vi "ASTI FREQ CALC v3.1 .vi"(8 "Calculate":bool, 9 "Path":u16(ring) items=["AMC 8 PRI : 7(A)", "AMC 8 PRI : 9(B)", "G13 ALT : 17(A)", "G13 ALT : 1(B)"], 10 "Input Frequency (MHz)":dbl=70.0 format="%.4g") -> (1 "C-band RX":dbl format="%.4g", 2 "C-Band TX":dbl format="%.4g")   [LabVIEW 2015]
uses:
  <vilib>/printing/EasyPrintingControls.llb/contents.ctl
  <vilib>/printing/EasyPrintingControls.llb/layout_options.ctl
  <vilib>/printing/EasyPrintingControls.llb/orientation.ctl
  <vilib>/printing/EasyPrintingControls.llb/panel_scaling_for_page.ctl
  <vilib>/printing/EasyPrintingControls.llb/margins.ctl
  <vilib>/printing/EasyPrintingControls.llb/margin_values.ctl
  <vilib>/printing/EasyPrintingControls.llb/measurement_system.ctl
  <vilib>/printing/EasyPrintingControls.llb/printer_options.ctl
  <vilib>/printing/EasyPrintingControls.llb/printing_method.ctl
  <vilib>/printing/EasyPrintingControls.llb/color_or_monochrome.ctl
  <vilib>/printing/EasyPrintingControls.llb/page_header_options.ctl
  <vilib>/printing/EasyPrintingControls.llb/page_headers.ctl
  <vilib>/printing/EasyPrintingControls.llb/page_header_content_options.ctl
  <vilib>/printing/EasyPrintingControls.llb/report_type.ctl
  <vilib>/Utility/file.llb/Read Delimited Spreadsheet (string).vi
  <vilib>/printing/EasyPrinting.llb/Easy Print VI Panel or Documentation (path).vi
  <vilib>/Utility/NIReport.llb/NI_ReportGenerationCore.lvlib
panel:
  in  "Print":bool
  out "TIME":string
  out "DATE":string
  out "Status":string
  in  "stop":bool
  in  "Tab Control":T1(tab)
  in  "Direction (L-Band Only)":u16(ring) items=["L-Band TX", "L-Band RX"]
  in  "Add to report":bool
  out "Frequency Ranges (Center)":string[][](array[string])
  out "70 2":dbl format="%.4g"
  out "70":dbl format="%.4g"
  out "L-RX":dbl format="%.4g"
  out "L-TX":dbl format="%.4g"
  in  "Clear":bool
  in  "Carrier":string[][](array[string])=[["Carrier/Link", "C-Band TX            ", "C-Band RX       ", "L-Band TX       ", "L-Band RX       ", "70MHz-IF     "], ["", "3840.000000", "1165.000000", "1310.000000", "70.000000", ""], ["", "0.000000", "0.000000", "0.000000", "0.000000", ""], ["", "3840.000000", "1165.000000", "1310.000000", "70.000000", ""], ["", "", "", "", "", ""], ["", "", "", "", "", ""], ["", "", "", "", "", ""], ["", "", "", "", "", ""], ["", "     ", "", "       ", "", ""], ["", "        ", "", "        ", "", ""]]
  out "Frequencies":string[][](array[string])=[["C-Band TX            ", "C-Band RX       ", "L-Band TX       ", "L-Band RX       ", "70MHz-IF     ", ""], ["", "", "", "", "", ""], ["", "", "", "", "", ""], ["", "", "", "", "", ""], ["", "", "", "", "", ""], ["", "", "", "", "", ""], ["", "     ", "", "       ", "", ""], ["", "        ", "", "        ", "", ""]]
  in  "Site":string
  # "ASTI FREQUENCY CALC"
  # "Transmit IF"
  # "70MHz"
  # "RF\nEquip"
  # "Transmitting\nModem"
  # "Or"
  # "L-Band"
  # "BUC LO = 4900"
  # "LO = 2225 MHz"
  # "All frequency values are in MHz"
  # "Sat"
  # "Receive IF"
  # "70MHz"
  # "RF\nEquip"
  # "Receiving\nModem"
  # "Or"
  # "Note: Downlink C-Band frequencies are not accessible at sites with L-Band IF\nIF/RF Equipment"
  # "L-Band"
  # "LNB LO = 5150"
  # "** Converters and modems are configured with 20 MHz offset at 70MHz-IF and converter CF"
  # "Edit carrier name\nprior to printing"
  # "For a single carrier"
  # "(LBand TX)  +  LBand RX = 2475 MHz"
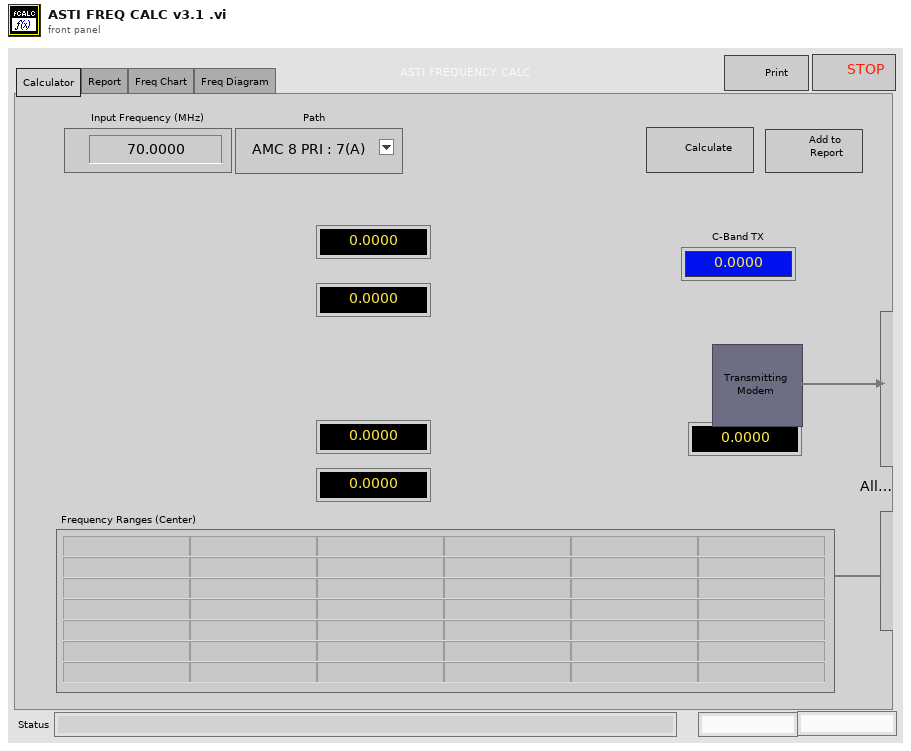
[diagram p1: front panel]
types:
  T1 = enum32{"Calculator", "Report", "Freq Chart", "Freq Diagram"}
  T2 = cluster{"C-Band TX":dbl, "C-band RX":dbl, "L-TX":dbl, "L-RX":dbl, "70":dbl}
  T3 = typedef "NI_ReportGenerationCore.lvlib/layout_options.ctl" = cluster{"orientation (unchanged)":T4, "panel scaling for page (unchanged)":T5, "margins":T6, "printer options":T9, "page header options":T12}
  T4 = typedef "NI_ReportGenerationCore.lvlib/orientation.ctl" = u16
  T5 = typedef "NI_ReportGenerationCore.lvlib/panel_scaling_for_page.ctl" = u16
  T6 = typedef "NI_ReportGenerationCore.lvlib/margins.ctl" = cluster{"override VI margins (false)":bool, "margins (1.00)":T7, "measurement system (default)":T8}
  T7 = typedef "NI_ReportGenerationCore.lvlib/margin_values.ctl" = cluster{"top":dbl, "left":dbl, "right":dbl, "bottom":dbl}
  T8 = typedef "NI_ReportGenerationCore.lvlib/measurement_system.ctl" = u16
  T9 = typedef "NI_ReportGenerationCore.lvlib/printer_options.ctl" = cluster{"destination printer name (current)":string, "printing method (unchanged)":T10, "color or monochrome (unchanged)":T11}
  T10 = typedef "NI_ReportGenerationCore.lvlib/printing_method.ctl" = u16
  T11 = typedef "NI_ReportGenerationCore.lvlib/color_or_monochrome.ctl" = u16
  T12 = typedef "NI_ReportGenerationCore.lvlib/page_header_options.ctl" = cluster{"page headers (unchanged)":T13, "page header content options":T14}
  T13 = typedef "NI_ReportGenerationCore.lvlib/page_headers.ctl" = u16
  T14 = typedef "NI_ReportGenerationCore.lvlib/page_header_content_options.ctl" = cluster{"Include VI Name":bool, "Include VI Path":bool, "Include Last Modification Date":bool, "Include Date Printed":bool, "Include Page Number":bool, "Include VI Icon":bool}
  T15 = typedef "NI_ReportGenerationCore.lvlib/report_type.ctl" = u16
  T16 = typedef "NI_ReportGenerationCore.lvlib/contents.ctl" = u16
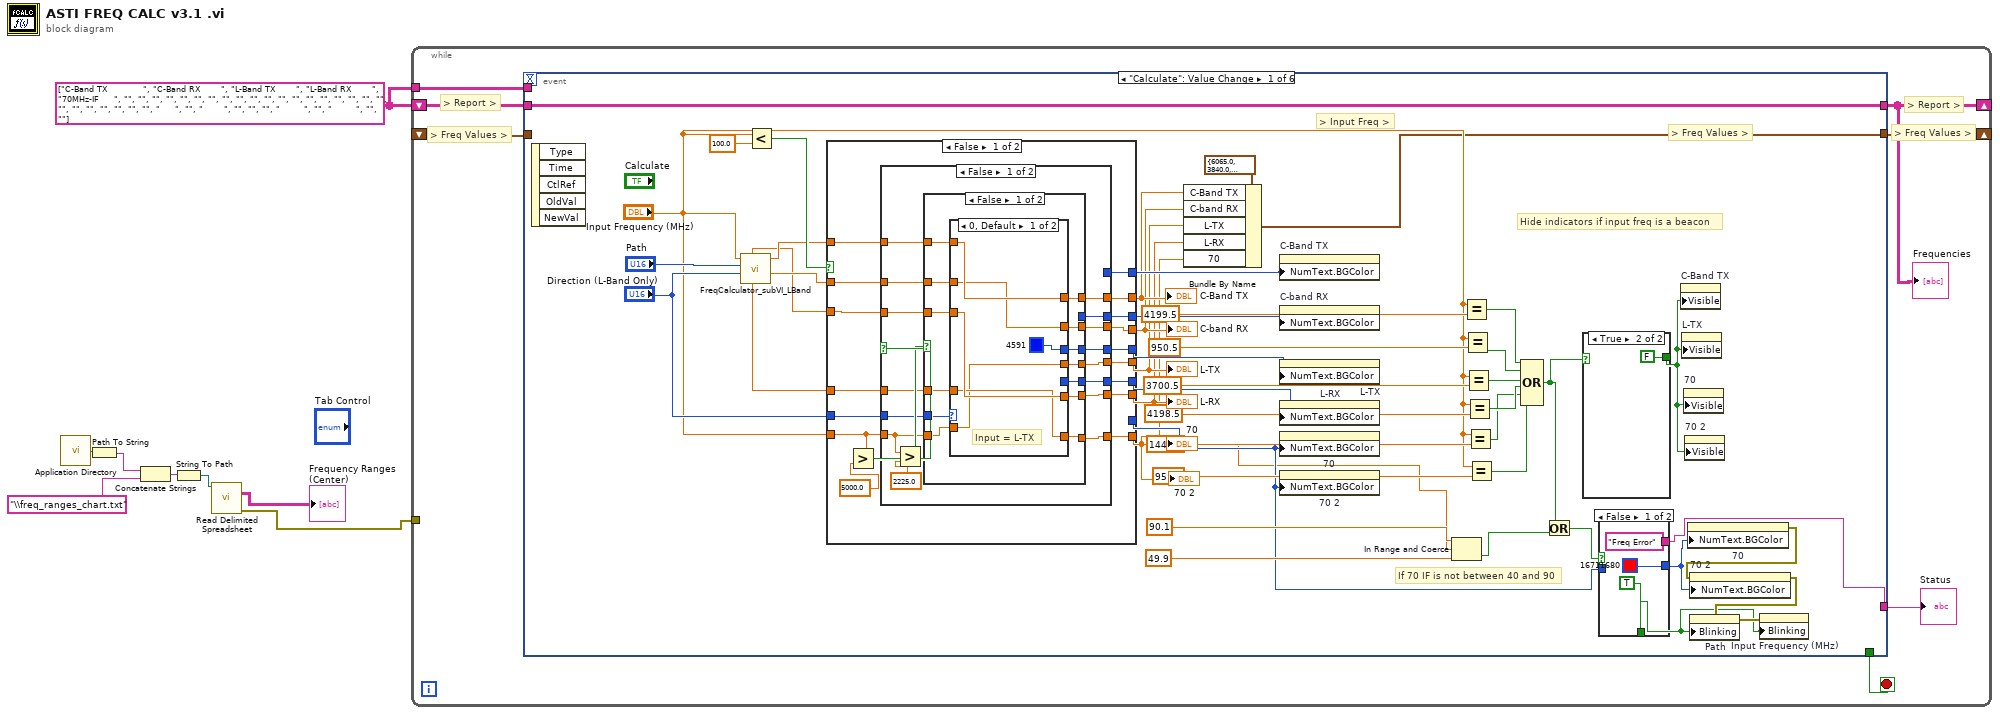
[diagram p0: block diagram]
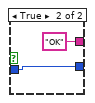
[diagram p2: hidden frame]
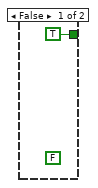
[diagram p3: hidden frame]
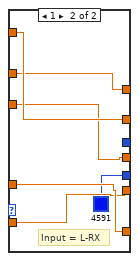
[diagram p4: hidden frame]
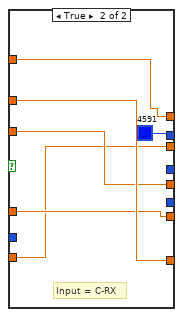
[diagram p5: hidden frame]
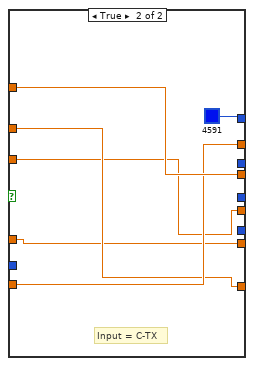
[diagram p6: hidden frame]
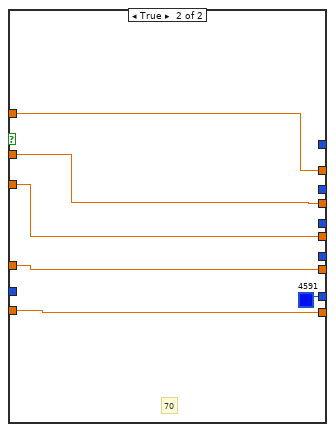
[diagram p7: hidden frame]
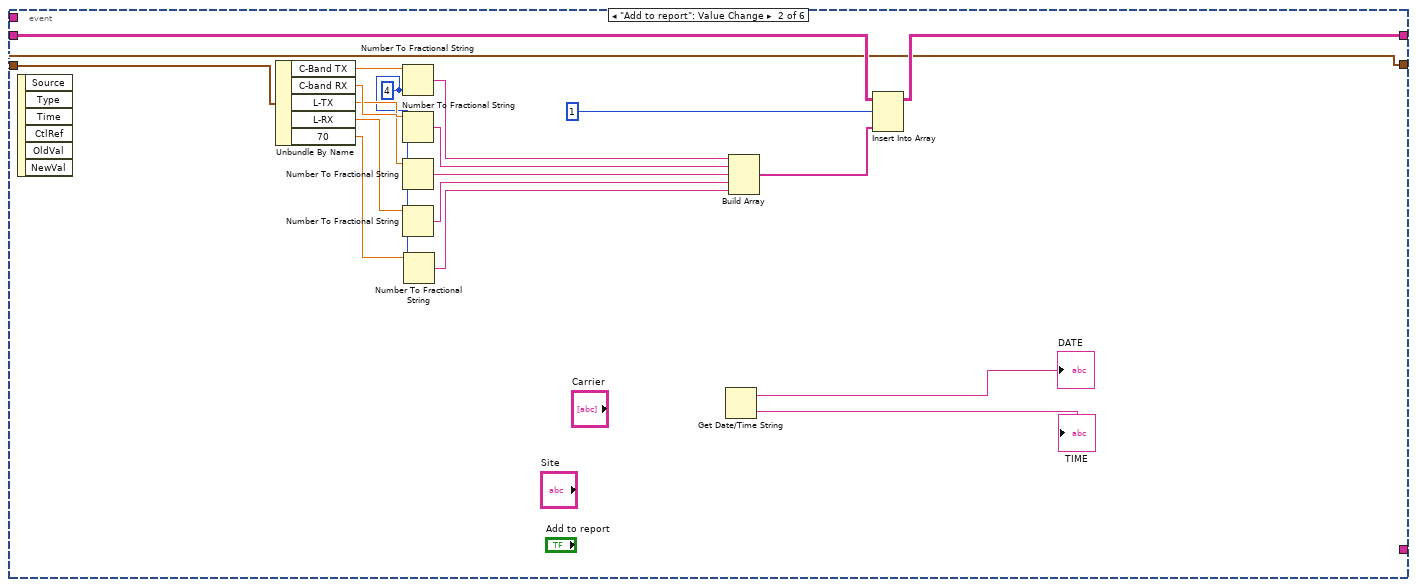
[diagram p8: hidden frame]
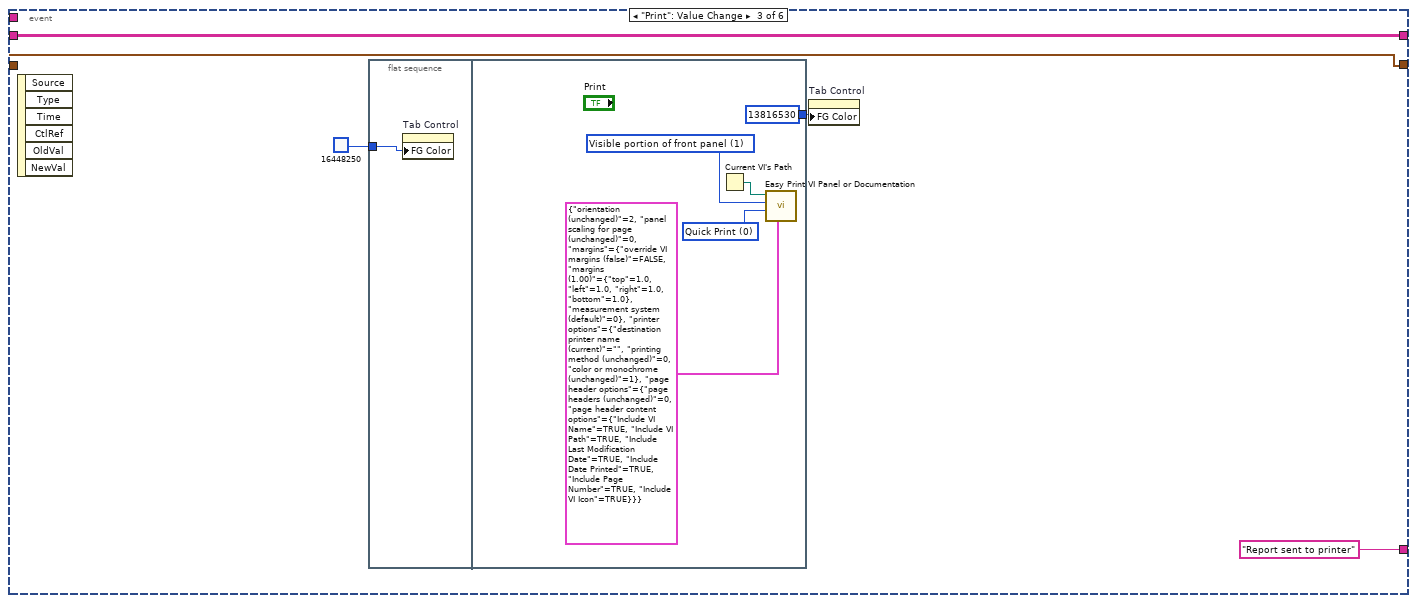
[diagram p9: hidden frame]
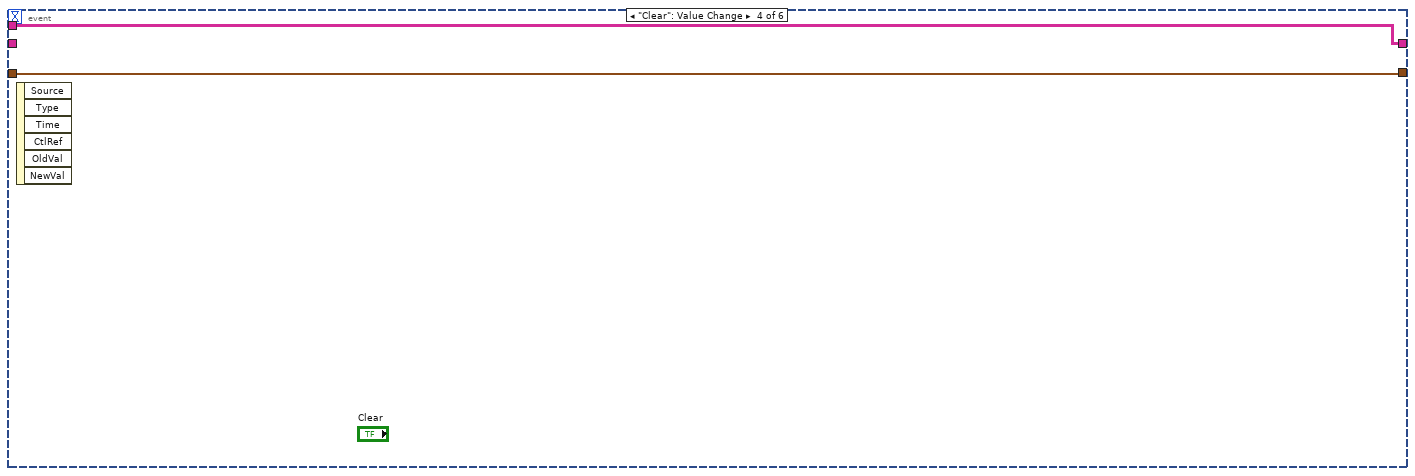
[diagram p10: hidden frame]
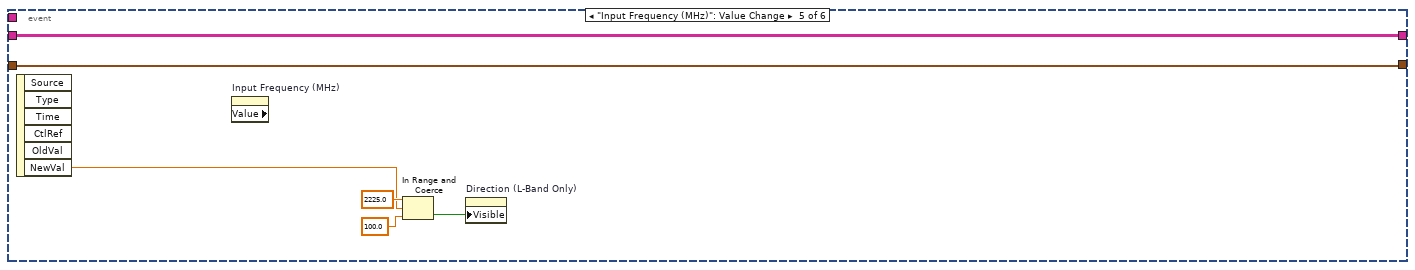
[diagram p11: hidden frame]
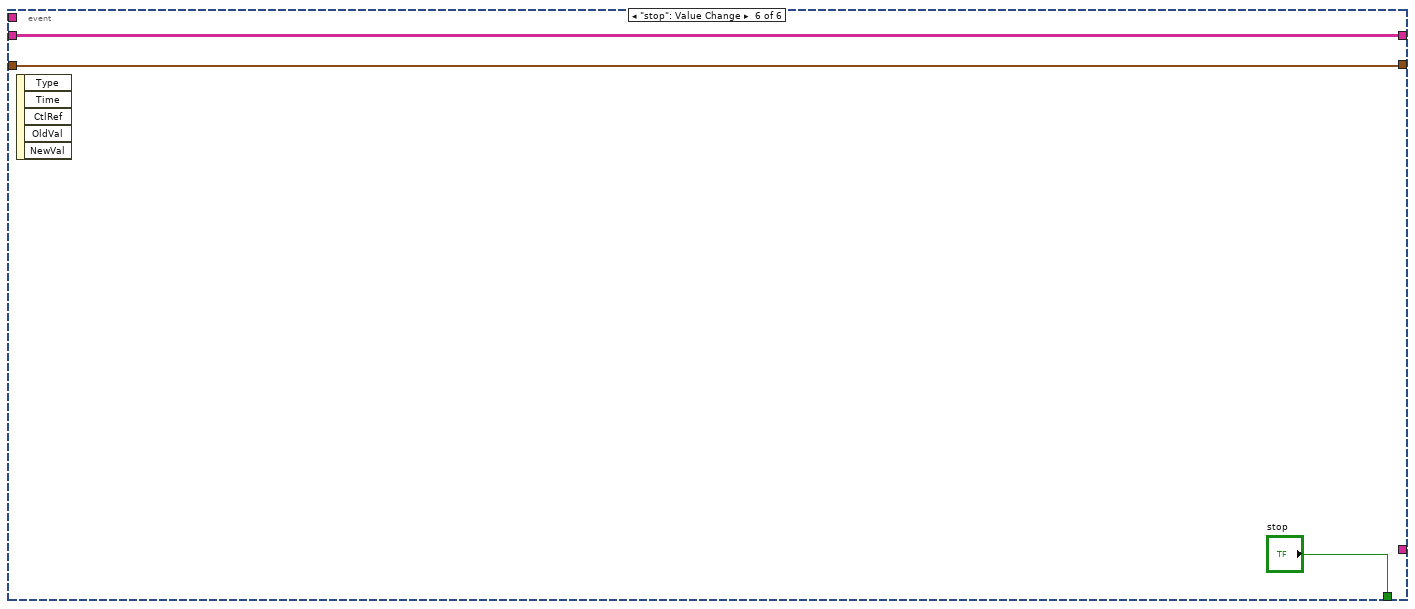
[diagram p12: hidden frame]
diagram:
  w1 = string[][] [["C-Band TX            ", "C-Band RX       ", "L-Band TX       ", "L-Band RX       ", "70MHz-IF     ", ""], ["", "", "", "", "", ""], ["", "", "", "", "", ""], ["", "", "", "", "", ""], ["", "", "", "", "", ""], ["", "     ", "", "       ", "", ""], ["", "        ", "", "        ", "", ""]] ("Frequency Report")
  n1 = call <vilib>:"Application Directory.vi"() -> ("Application Directory"=w7:path)
  n2 = Path To String(path=w7) -> (string=w5:string)
  n3 = Concatenate Strings(w5, "\\freq_ranges_chart.txt") -> (w4:string)
  n4 = String To Path(string=w4) -> (path=w3:path)
  n5 = call-poly <vilib>:"Read Delimited Spreadsheet.vi"("file path (dialog if empty)"=w3) -> ("all rows"=→"Frequency Ranges (Center)":string[][], "error out"=w2:errorcluster)  [unwired: 9 in, 4 out]
  n6 = while {
    tunnel: w2 -> [_]
    shift-right: [w14] -> _
    shift-left: _ -> [w13]
    shift-right: [w10] -> _
    shift-left: w1 -> [w12]
    tunnel: w1 -> [w9]
    stop <- w15 stop-if-true
    # "> Report >"
    # "> Report >"
    # "> Freq Values >"
    # "> Freq Values >"
    n7 = event shown="[0] \"Calculate\": Value Change" {
      selector: _ -> [_ _ _ _ _ _]
      dyn-events: _ -> [_ _ _ _ _ _]
      timeout: _ -> [_ _ _ _ _ _]
      tunnel: [_ _ _ _ _ "stop"] -> w15
      tunnel: [w18 w148 w163 w174 w176 w182] -> w14
      tunnel: w13 -> [_ w148 w163 w174 w176 w182]
      tunnel: w12 -> [w17 w152 w164 _ w177 w183]
      tunnel: [w17 w149 w164 w175 w177 w183] -> w10
      tunnel: [w16 _ "Report sent to printer" ("Status") _ _ _] -> w11
      tunnel: w9 -> [_ _ _ w175 _ _]
      event "Calculate": Value Change {
        # "> Freq Values >"
        # "> Input Freq >"
        # "If 70 IF is not between 40 and 90"
        # "Hide indicators if input freq is a beacon"
        n8 = event-data() -> ()  [unwired: 1 in, 5 out]
        n9 = call "FreqCalculator_subVI_LBand.vi"("Direction (L-Band Only)"="Direction (L-Band Only)", "Path"="Path", "Input Frequency"="Input Frequency (MHz)") -> ("Out2"=w57:dbl, "Out1"=w58:dbl, "Out 4"=w55:dbl, "Out 3"=w56:dbl)  [unwired: 1 in, 4 out]
        n10 = Less?(x="Input Frequency (MHz)", y=100.0) -> (x < y?=w59:bool)
        n11 = case shown="False" w59 {
          tunnel: [w81 w144] -> w24
          tunnel: w58 -> [w82 w144]
          tunnel: [w83 w143] -> w22
          tunnel: w57 -> [w78 w143]
          tunnel: w56 -> [w77 w142]
          tunnel: [w75 w142] -> w21
          tunnel: w55 -> [w74 w141]
          tunnel: [w76 w141] -> w20
          tunnel: "Input Frequency (MHz)" -> [w80 w140]
          tunnel: [w79 w140] -> w19
          tunnel: "Direction (L-Band Only)" -> [w73 _]
          tunnel: [w72 _] -> w50
          tunnel: [w71 _] -> w53
          tunnel: [w70 _] -> w52
          tunnel: [w69 _] -> w51
          tunnel: [_ u32 4591] -> w25
          frame False {
            n12 = Greater?(x=w80, y=5000.0) -> (0:w84:bool)
            n13 = case shown="False" w84 {
              tunnel: [w90 w138] -> w83
              tunnel: w82 -> [w98 w138]
              tunnel: [w99 w137] -> w81
              tunnel: w80 -> [w89 w137]
              tunnel: [w97 w136] -> w79
              tunnel: w78 -> [w96 w136]
              tunnel: [w93 w134] -> w76
              tunnel: w77 -> [w94 w135]
              tunnel: [w95 w135] -> w75
              tunnel: w74 -> [w92 w134]
              tunnel: w73 -> [w91 _]
              tunnel: [_ u32 4591] -> w72
              tunnel: [w88 _] -> w71
              tunnel: [w87 _] -> w70
              tunnel: [w86 _] -> w69
              frame False {
                n14 = Greater?(x=w89, y=2225.0) -> (0:w100:bool)
                n15 = case shown="False" w100 {
                  tunnel: [w111 w132] -> w99
                  tunnel: w98 -> [w113 w132]
                  tunnel: [w106 w131] -> w97
                  tunnel: w96 -> [w110 w131]
                  tunnel: [w109 w130] -> w95
                  tunnel: w94 -> [w108 w130]
                  tunnel: [w104 w129] -> w93
                  tunnel: w92 -> [w107 w129]
                  tunnel: w91 -> [w114 _]
                  tunnel: [w112 w128] -> w90
                  tunnel: w89 -> [w105 w128]
                  tunnel: [w103 _] -> w88
                  tunnel: [w102 _] -> w87
                  tunnel: [_ u32 4591] -> w86
                  frame False {
                    n16 = case shown="0, Default" w114 {
                      tunnel: w113 -> [w120 w126]
                      tunnel: [w119 w126] -> w112
                      tunnel: [w120 w125] -> w111
                      tunnel: w110 -> [w119 w125]
                      tunnel: [w116 w124] -> w109
                      tunnel: w108 -> [w118 w124]
                      tunnel: [w117 w123] -> w106
                      tunnel: w107 -> [w117 w123]
                      tunnel: [w118 w122] -> w104
                      tunnel: w105 -> [w116 w122]
                      tunnel: [_ u32 4591] -> w103
                      tunnel: [u32 4591 _] -> w102
                      frame 0, Default {
                        # "Input = L-TX"
                      }
                      frame 1 {
                        # "Input = L-RX"
                      }
                    }
                  }
                  frame True {
                    # "Input = C-RX"
                  }
                }
              }
              frame True {
                # "Input = C-TX"
              }
            }
          }
          frame True {
            # "70"
          }
        }
        "C-Band TX" <- w24
        "C-band RX" <- w22
        "L-TX" <- w21
        "L-RX" <- w20
        "70" <- w19
        "70 2" <- w19
        n17 = Bundle By Name(cluster=T2 {"C-Band TX"=6065.0, "C-band RX"=3840.0, "L-TX"=1165.0, "L-RX"=1310.0, "70"=70.0} ("input cluster"), "C-Band TX"=w24, "C-band RX"=w22, "L-TX"=w21, "L-RX"=w20, "70"=w19) -> (w18:T2)
        n18 = property on="C-Band TX" class="DigNum (strict)"("NumText.BGColor"=w50) -> ()  [unwired: 2 in, 2 out]
        n19 = property on="C-band RX" class="DigNum (strict)"("NumText.BGColor"=w51) -> ()  [unwired: 2 in, 2 out]
        n20 = property on="L-TX" class="DigNum (strict)"("NumText.BGColor"=w52) -> ()  [unwired: 2 in, 2 out]
        n21 = property on="L-RX" class="DigNum (strict)"("NumText.BGColor"=w53) -> ()  [unwired: 2 in, 2 out]
        n22 = property on="70" class="DigNum (strict)"("NumText.BGColor"=w25) -> ()  [unwired: 2 in, 2 out]
        n23 = property on="70 2" class="DigNum (strict)"("NumText.BGColor"=w25) -> ()  [unwired: 2 in, 2 out]
        n24 = In Range and Coerce(upper limit=90.1, x=w19, lower limit=49.9) -> (In Range?=w27:bool)  [unwired: 1 out]
        n25 = Equal?(x="Input Frequency (MHz)", y=4199.5) -> (x = y?=w44:bool)
        n26 = Equal?(x="Input Frequency (MHz)", y=950.5) -> (x = y?=w43:bool)
        n27 = Equal?(x="Input Frequency (MHz)", y=3700.5) -> (x = y?=w42:bool)
        n28 = Equal?(x="Input Frequency (MHz)", y=4198.5) -> (x = y?=w41:bool)
        n29 = Equal?(x="Input Frequency (MHz)", y=1449.5) -> (x = y?=w40:bool)
        n30 = Equal?(x="Input Frequency (MHz)", y=951.5) -> (x = y?=w37:bool)
        n31 = Compound Arithmetic op=OR(w44, w43, w42, w41, w40, w37) -> (w28:bool)
        n32 = Or(x=w28, y=w27) -> (x .or. y?=w26:bool)
        n33 = case shown="True" w28 {
          tunnel: [TRUE FALSE] -> w29
          frame False {
            (unwired) FALSE ("Blinking")
          }
          frame True {
          }
        }
        n34 = case shown="False" w26 {
          tunnel: [u32 16711680 w66] -> w31
          tunnel: [TRUE ("Blinking") _] -> w30
          tunnel: w25 -> [_ w66]
          tunnel: ["Freq Error" ("Status") "OK" ("Status")] -> w16
          frame False {
          }
          frame True {
          }
        }
        n35 = property on="C-Band TX" class="DigNum (strict)"("Visible"=w29) -> ()  [unwired: 2 in, 2 out]
        n36 = property on="L-TX" class="DigNum (strict)"("Visible"=w29) -> ()  [unwired: 2 in, 2 out]
        n37 = property on="70" class="DigNum (strict)"("Visible"=w29) -> ()  [unwired: 2 in, 2 out]
        n38 = property on="70 2" class="DigNum (strict)"("Visible"=w29) -> ()  [unwired: 2 in, 2 out]
        n39 = property on="70" class="DigNum (strict)"("NumText.BGColor"=w31) -> (error out=w34:errorcluster)  [unwired: 2 in, 1 out]
        n40 = property on="70 2" class="DigNum (strict)"(error in=w34, "NumText.BGColor"=w31) -> (error out=w32:errorcluster)  [unwired: 1 in, 1 out]
        n41 = property on="Path" class="Ring (strict)"(error in=w32, "Blinking"=w30) -> (error out=w33:errorcluster)  [unwired: 1 in, 1 out]
        n42 = property on="Input Frequency (MHz)" class="DigNum (strict)"(error in=w33, "Blinking"=w30) -> ()  [unwired: 1 in, 2 out]
      }
      event "Add to report": Value Change {
        w145 = i16 4 ("precision (6)")
        n43 = event-data() -> ()  [unwired: 1 in, 6 out]
        n44 = Unbundle By Name(w148) -> ("C-Band TX"=w162:dbl, "C-band RX"=w161:dbl, "L-TX"=w160:dbl, "L-RX"=w159:dbl, "70"=w158:dbl)
        n45 = Number To Fractional String(number=w162, precision (6)=w145) -> (F-format string=w157:string)  [unwired: 2 in]
        n46 = Number To Fractional String(number=w161, precision (6)=w145) -> (F-format string=w156:string)  [unwired: 2 in]
        n47 = Number To Fractional String(number=w160, precision (6)=w145) -> (F-format string=w155:string)  [unwired: 2 in]
        n48 = Number To Fractional String(number=w159, precision (6)=w145) -> (F-format string=w154:string)  [unwired: 2 in]
        n49 = Number To Fractional String(number=w158, precision (6)=w145) -> (F-format string=w153:string)  [unwired: 2 in]
        n50 = Get Date/Time String() -> (date string=→"DATE":string, time string=→"TIME":string)  [unwired: 3 in]
        n51 = Build Array(w157, w156, w155, w154, w153) -> (w151:string[])
        n52 = Insert Into Array(array=w152, index (row)=1, new element=w151) -> (w149:string[][])  [unwired: 1 in]
      }
      event "Print": Value Change {
        n53 = event-data() -> ()  [unwired: 1 in, 6 out]
        n54 = flat-sequence {
          tunnel: u32 16448250 -> [w168]
          tunnel: [u32 13816530 ("Colors:BG Color")] -> w166
          frame #0 {
            n55 = property on="Tab Control" class="TabCtl (strict)"("FG Color"=w168) -> ()  [unwired: 2 in, 2 out]
          }
          frame #1 {
            w170 = T15 0 items=["Quick Print", "Standard Report", "HTML", "Word", "Excel"] ("report type (Quick Print)")
            w173 = T16 1 items=["Complete front panel", "Visible portion of front panel", "Icon, description, panel and diagram", "Documentation: Using the panel", "Documentation: Using as a subVI", "Documentation: Complete", "Documentation: Custom"] ("contents (complete front panel)")
            n56 = Current VI's Path() -> (path=w172:path)
            n57 = call-poly <vilib>:"Easy Print VI Panel or Documentation.vi"("layout options"=T3 {"orientation (unchanged)"=2, "panel scaling for page (unchanged)"=0, "margins"={"override VI margins (false)"=FALSE, "margins (1.00)"={"top"=1.0, "left"=1.0, "right"=1.0, "bottom"=1.0}, "measurement system (default)"=0}, "printer options"={"destination printer name (current)"="", "printing method (unchanged)"=0, "color or monochrome (unchanged)"=1}, "page header options"={"page headers (unchanged)"=0, "page header content options"={"Include VI Name"=TRUE, "Include VI Path"=TRUE, "Include Last Modification Date"=TRUE, "Include Date Printed"=TRUE, "Include Page Number"=TRUE, "Include VI Icon"=TRUE}}}, "report type (Quick Print)"=w170, "contents (complete front panel)"=w173, "VI path"=w172) -> ()  [unwired: 6 in, 2 out]
          }
        }
        n58 = property on="Tab Control" class="TabCtl (strict)"("FG Color"=w166) -> ()  [unwired: 2 in, 2 out]
      }
      event "Clear": Value Change {
        n59 = event-data() -> ()  [unwired: 1 in, 6 out]
      }
      event "Input Frequency (MHz)": Value Change {
        n60 = event-data() -> ("NewVal"=w178:dbl)  [unwired: 1 in, 5 out]
        n61 = property on="Input Frequency (MHz)" class="DigNum (strict)" props=["Value"]() -> ()  [unwired: 2 in, 3 out]
        n62 = In Range and Coerce(upper limit=2225.0, x=w178, lower limit=100.0) -> (In Range?=w179:bool)  [unwired: 1 out]
        n63 = property on="Direction (L-Band Only)" class="Ring (strict)"("Visible"=w179) -> ()  [unwired: 2 in, 2 out]
      }
      event "stop": Value Change {
        n64 = event-data() -> ()  [unwired: 1 in, 5 out]
      }
    }
    "Status" <- w11
    "Frequencies" <- w10
  }
